vi "2015 Open Close Reference.vi"(7 "Byte Stream File in":refnum<file>, 8 "error in (no error)":errorcluster, 10 "New File?":bool) -> (0 "error out":errorcluster, 3 "String":string)   [LabVIEW 2014]
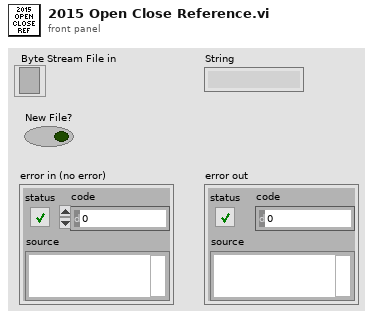
[diagram p1: front panel]
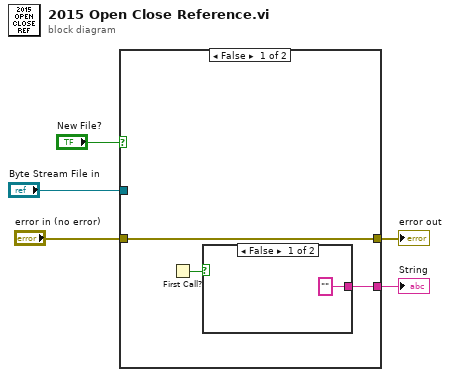
[diagram p0: block diagram]
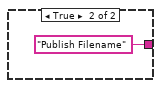
[diagram p2: hidden frame]
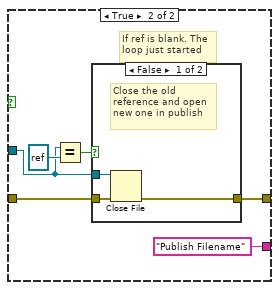
[diagram p3: hidden frame]
diagram:
  n1 = case shown="False" "New File?" {
    tunnel: [w8 "Publish Filename"] -> w1
    tunnel: "Byte Stream File in" -> [_ w13]
    tunnel: "error in (no error)" -> [w7 w12]
    tunnel: [w7 w11] -> w3
    frame False {
      n2 = First Call?() -> (First Call?: T/F=w6:bool)
      n3 = case shown="False" w6 {
        tunnel: ["" "Publish Filename"] -> w8
        frame False {
        }
        frame True {
        }
      }
    }
    frame True {
      # "If ref is blank. The\nloop just started"
      n4 = Equal?(x=w13, y=refnum<file> refnum ("Blank")) -> (x = y?=w14:bool)
      n5 = case shown="False" w14 {
        tunnel: w13 -> [w19 _]
        tunnel: w12 -> [w18 w20]
        tunnel: [w17 w20] -> w11
        frame False {
          # "Close the old\nreference and open\nnew one in publish"
          n6 = Close File(refnum=w19, error in=w18) -> (error out=w17:errorcluster)  [unwired: 1 out]
        }
        frame True {
        }
      }
    }
  }
  "error out" <- w3
  "String" <- w1
